vi "GUI.Stream.Disable.vi"(8 "error in (no error)":errorcluster, 11 "State Variables in":T1) -> (0 "error out":errorcluster)   [LabVIEW 2025, in "XNET Bus Monitor Client.lvlib"]
uses:
  XNET Bus Monitor Client.lvlib
  Types/GUI.StateVariables.ctl
  Types/GUI.Controls.Refs.ctl
  bus_monitor_client/RPC Messages/ni_bus_monitor_api_DirectionFilter.ctl
  bus_monitor_client/RPC Messages/ni_bus_monitor_api_FrameFilter.ctl
  Types/StreamEngine.QueueRefs.ctl
  Types/StreamEngine.CmdQueueData.ctl
  Types/StreamEngine.CmdQueueData.Cmd.ctl
  Types/SubProcessEngine.QueueRefs.ctl
  Types/SubProcessEngine.CmdQueueData.ctl
  Types/SubProcessEngine.CmdQueueData.Cmd.ctl
  Types/gRPC.ConnectionInfo.ctl
  <vilib>/gRPC/LabVIEW gRPC Library/Shared/grpcId.ctl
  bus_monitor_client/RPC Messages/ni_bus_monitor_api_Session.ctl
  <vilib>/Utility/miscctls.llb/LVRowAndColumnUnsignedTypeDef.ctl
  <vilib>/gRPC/LabVIEW gRPC Library/grpc-lvsupport-release.lvlib
  bus_monitor_client/bus_monitor_client.lvlib
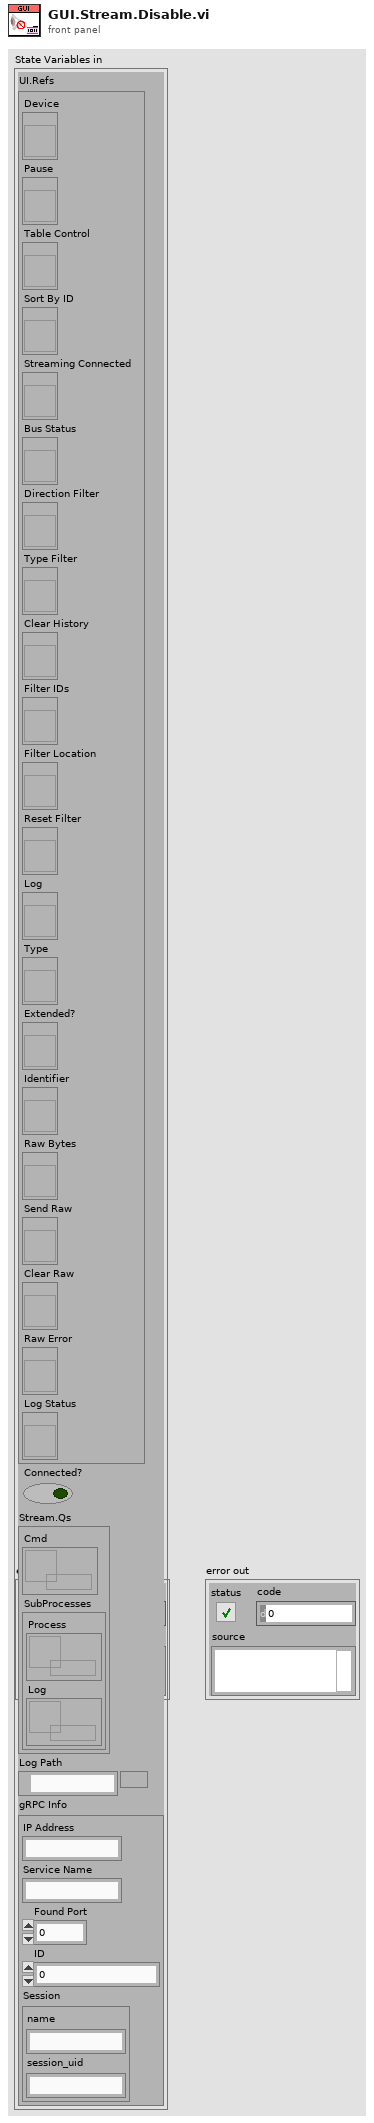
[diagram p1: front panel]
types:
  T1 = typedef "XNET Bus Monitor Client.lvlib/GUI.StateVariables.ctl" = cluster{"UI.Refs":T2, "Connected?":bool, "Stream.Qs":T3, "Log Path":path, "gRPC Info":T5}
  T2 = typedef "XNET Bus Monitor Client.lvlib/GUI.Controls.Refs.ctl" = cluster{"Device":refnum<vi>, "Pause":refnum<vi>, "Table Control":refnum<vi>, "Sort By ID":refnum<vi>, "Streaming Connected":refnum<vi>, "Bus Status":refnum<vi>, "Direction Filter":refnum<vi>, "Type Filter":refnum<vi>, "Clear History":refnum<vi>, "Filter IDs":refnum<vi>, "Filter Location":refnum<vi>, "Reset Filter":refnum<vi>, "Log":refnum<vi>, "Type":refnum<vi>, "Extended?":refnum<vi>, "Identifier":refnum<vi>, "Raw Bytes":refnum<vi>, "Send Raw":refnum<vi>, "Clear Raw":refnum<vi>, "Raw Error":refnum<vi>, "Log Status":refnum<vi>}
  T3 = typedef "XNET Bus Monitor Client.lvlib/StreamEngine.QueueRefs.ctl" = cluster{"Cmd":refnum<queue>, "SubProcesses":T4}
  T4 = typedef "XNET Bus Monitor Client.lvlib/SubProcessEngine.QueueRefs.ctl" = cluster{"Process":refnum<queue>, "Log":refnum<queue>}
  T5 = typedef "XNET Bus Monitor Client.lvlib/gRPC.ConnectionInfo.ctl" = cluster{"IP Address":string, "Service Name":string, "Found Port":u64, "ID":T6, "Session":T7}
  T6 = typedef "grpc-lvsupport-release.lvlib/grpcId.ctl" = u64
  T7 = typedef "bus_monitor_client.lvlib/ni_bus_monitor_api_Session.ctl" = cluster{"name":string, "session_uid":string}
  T8 = enum16{"CAN Data", "CAN Remote", "CAN Bus Error", "CAN 2.0 Data", "CAN FD Data", "CAN FD+BRS Data", "J1939 Data", "Delay", "Log Trigger", "Start Trigger"}
  T9 = typedef "LVRowAndColumnUnsignedTypeDef.ctl" = cluster{"Row":u32, "Column":u32}
  T10 = enum8{"Enabled", "Disabled", "Disabled and Grayed Out"}
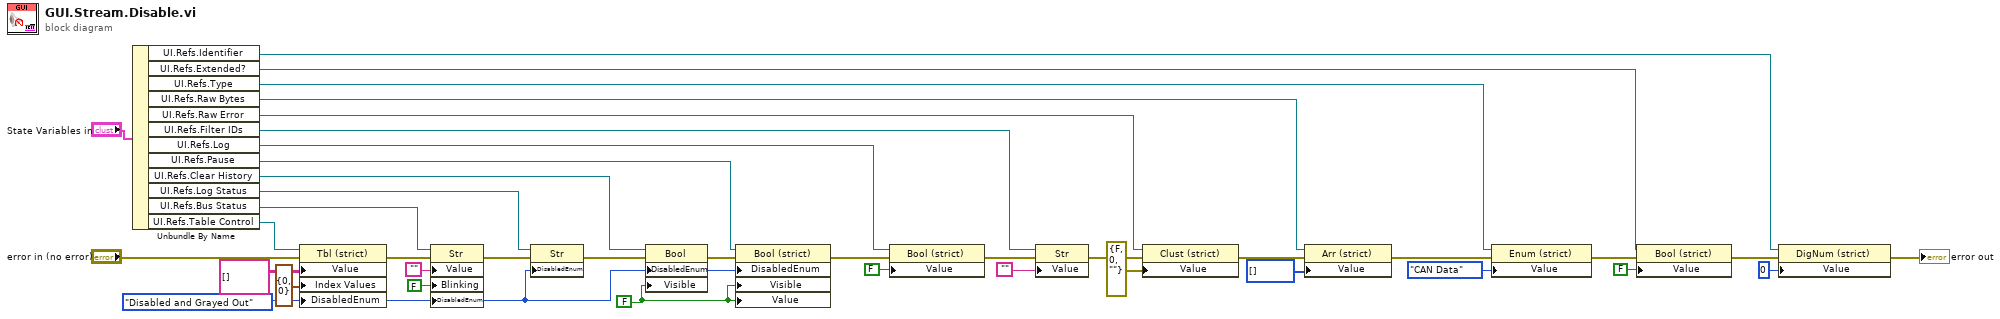
[diagram p0: block diagram]
diagram:
  w29 = FALSE ("Value")
  w3 = T10."Disabled and Grayed Out" ("Disabled")
  n1 = Unbundle By Name("State Variables in") -> ("UI.Refs.Identifier"=w13:refnum<vi>, "UI.Refs.Extended?"=w15:refnum<vi>, "UI.Refs.Type"=w17:refnum<vi>, "UI.Refs.Raw Bytes"=w20:refnum<vi>, "UI.Refs.Raw Error"=w21:refnum<vi>, "UI.Refs.Filter IDs"=w23:refnum<vi>, "UI.Refs.Log"=w27:refnum<vi>, "UI.Refs.Pause"=w30:refnum<vi>, "UI.Refs.Clear History"=w32:refnum<vi>, "UI.Refs.Log Status"=w4:refnum<vi>, "UI.Refs.Bus Status"=w36:refnum<vi>, "UI.Refs.Table Control"=w38:refnum<vi>)
  n2 = property class="Tbl (strict)"(reference=w38, error in="error in (no error)", "Value"=string[][] [], "Index Values"=T9 {"Row"=0, "Column"=0}, "DisabledEnum"=w3) -> (error out=w5:errorcluster)  [unwired: 1 out]
  n3 = property class="Str"(reference=w36, error in=w5, "Value"="", "Blinking"=FALSE, "DisabledEnum"=w3) -> (error out=w2:errorcluster)  [unwired: 1 out]
  n4 = property class="Str"(reference=w4, error in=w2, "DisabledEnum"=w3) -> (error out=w1:errorcluster)  [unwired: 1 out]
  n5 = property class="Bool"(reference=w32, error in=w1, "DisabledEnum"=w3, "Visible"=w29) -> (error out=w31:errorcluster)  [unwired: 1 out]
  n6 = property class="Bool (strict)"(reference=w30, error in=w31, "DisabledEnum"=w3, "Visible"=w29, "Value"=w29) -> (error out=w25:errorcluster)  [unwired: 1 out]
  n7 = property class="Bool (strict)"(reference=w27, error in=w25, "Value"=FALSE ("Visible")) -> (error out=w24:errorcluster)  [unwired: 1 out]
  n8 = property class="Str"(reference=w23, error in=w24, "Value"="") -> (error out=w19:errorcluster)  [unwired: 1 out]
  n9 = property class="Clust (strict)"(reference=w21, error in=w19, "Value"=errorcluster {"status"=FALSE, "code"=0, "source"=""}) -> (error out=w18:errorcluster)  [unwired: 1 out]
  n10 = property class="Arr (strict)"(reference=w20, error in=w18, "Value"=u8[] []) -> (error out=w16:errorcluster)  [unwired: 1 out]
  n11 = property class="Enum (strict)"(reference=w17, error in=w16, "Value"=T8."CAN Data") -> (error out=w14:errorcluster)  [unwired: 1 out]
  n12 = property class="Bool (strict)"(reference=w15, error in=w14, "Value"=FALSE) -> (error out=w12:errorcluster)  [unwired: 1 out]
  n13 = property class="DigNum (strict)"(reference=w13, error in=w12, "Value"=u32 0) -> (error out=→"error out":errorcluster)  [unwired: 1 out]
